vi "Build String.vi"(7 "Variables":refnum<class "Variables.lvclass">, 10 "error in (no error)":errorcluster, 11 "Format String in":refnum<class "Format String.lvclass">) -> (2 "error out":errorcluster, 3 "String":string)   [LabVIEW 2020, in "VolatusSeq.lvlib" / "Format String.lvclass"]
uses:
  Format String.lvclass
  Variables/Variables.lvclass
  Format String.lvclass/Format String.ctl
  Condition Value/Condition Value.lvclass/Condition Value.ctl
  lv-vecto/Vecto/Channel DBL/Channel DBL.lvclass/Channel DBL.ctl
  Variables/Variables.lvclass/Variables.ctl
  lv-vecto/Vecto/Channel DBL/Current Value.vi
  Variables/Get.vi
  lv-vecto/Vecto/Group DBL/Value by Index.vi
  Condition Value/Condition Value.lvclass
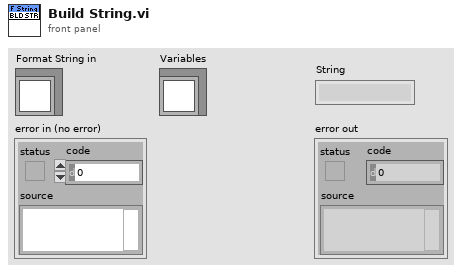
[diagram p1: front panel]
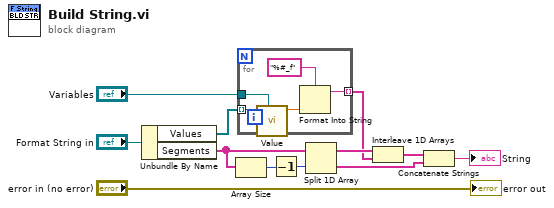
[diagram p0: block diagram]
diagram:
  n1 = Unbundle By Name("Format String in") -> ("Values"=w10:refnum<class "Condition Value.lvclass">[], "Segments"=w8:string[])
  n2 = Array Size(array=w8) -> (size(s)=w7:i32)
  n3 = for {
    tunnel: w10 -> [w17] mode=indexing
    tunnel: "Variables" -> [w16]
    tunnel: [w13] -> w4 mode=indexing
    n4 = call "Value.vi"("Variables"=w16, "Condition Value in"=w17) -> ("Value"=w15:dbl)  [unwired: 8 in, 1 out]
    n5 = Format Into String(format string="%#_f", w15) -> (resulting string=w13:string)  [unwired: 2 in, 1 out]
  }
  n6 = Decrement(x=w7) -> (x-1=w6:i32)
  n7 = Split 1D Array(array=w8, index=w6) -> (first subarray=w5:string[], second subarray=w2:string[])
  n8 = Interleave 1D Arrays(w5, w4) -> (w3:string[])
  n9 = Concatenate Strings(w3, w2) -> (→"String":string)
  "error out" <- "error in (no error)"
